vi "WriteXML.vi"(8 "error in (no error)":errorcluster, 10 "Path":path, 11 "PixelflySettings in":refnum<class "PixelflySettings.lvclass">) -> (0 "error out":errorcluster, 3 "PixelflySettings out":refnum<class "PixelflySettings.lvclass">)   [LabVIEW 2011, in "Tools.lvlib" / "Settings.lvlib" / "PixelflySettings.lvclass"]
uses:
  PixelflySettings.lvclass
  NativeXML/NativeXML.lvclass
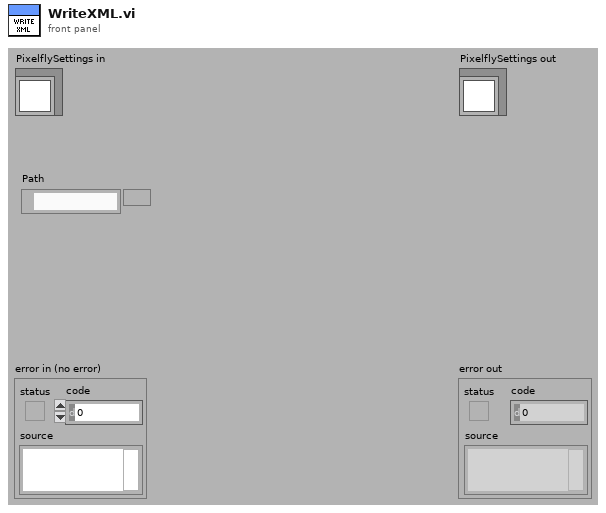
[diagram p1: front panel]
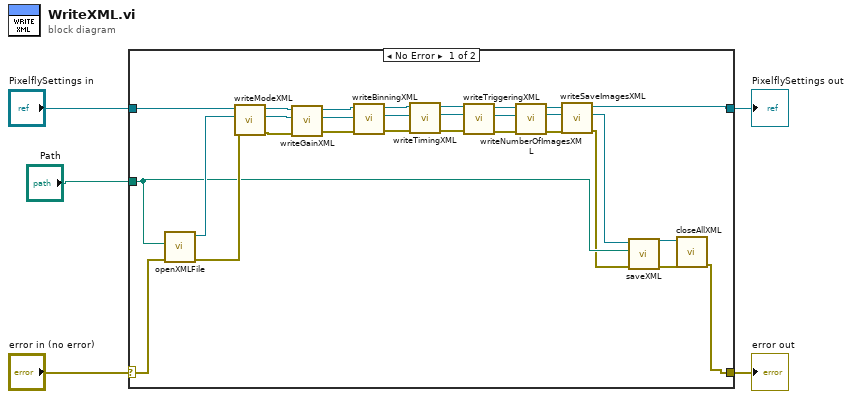
[diagram p0: block diagram]
diagram:
  n1 = case shown="No Error" "error in (no error)" {
    selector: "error in (no error)" -> [w19 w36]
    tunnel: [w15 w36] -> w4
    tunnel: [w8 w35] -> w2
    tunnel: "PixelflySettings in" -> [w34 w35]
    tunnel: "Path" -> [w18 _]
    frame No Error {
      n2 = call "openXMLFile.vi"("error in (no error)"=w19, "Path"=w18) -> ("error out"=w20:errorcluster, "NativeXML out"=w21:refnum<class "NativeXML.lvclass">)  [unwired: 8 in]
      n3 = call "writeModeXML.vi"("error in (no error)"=w20, "NativeXML in"=w21, "PixelflySettings in"=w34) -> ("error out"=w22:errorcluster, "NativeXML out"=w29:refnum<class "NativeXML.lvclass">, "PixelflySettings out"=w33:refnum<class "PixelflySettings.lvclass">)  [unwired: 6 in]
      n4 = call "writeGainXML.vi"("error in (no error)"=w22, "NativeXML in"=w29, "PixelflySettings in"=w33) -> ("error out"=w23:errorcluster, "NativeXML out"=w28:refnum<class "NativeXML.lvclass">, "PixelflySettings out"=w32:refnum<class "PixelflySettings.lvclass">)  [unwired: 6 in]
      n5 = call "writeBinningXML.vi"("error in (no error)"=w23, "NativeXML in"=w28, "PixelflySettings in"=w32) -> ("error out"=w24:errorcluster, "NativeXML out"=w27:refnum<class "NativeXML.lvclass">, "PixelflySettings out"=w31:refnum<class "PixelflySettings.lvclass">)  [unwired: 6 in]
      n6 = call "writeTimingXML.vi"("error in (no error)"=w24, "NativeXML in"=w27, "PixelflySettings in"=w31) -> ("error out"=w25:errorcluster, "NativeXML out"=w26:refnum<class "NativeXML.lvclass">, "PixelflySettings out"=w30:refnum<class "PixelflySettings.lvclass">)  [unwired: 6 in]
      n7 = call "writeTriggeringXML.vi"("error in (no error)"=w25, "NativeXML in"=w26, "PixelflySettings in"=w30) -> ("error out"=w14:errorcluster, "NativeXML out"=w13:refnum<class "NativeXML.lvclass">, "PixelflySettings out"=w12:refnum<class "PixelflySettings.lvclass">)  [unwired: 6 in]
      n8 = call "writeNumberOfImagesXML.vi"("error in (no error)"=w14, "NativeXML in"=w13, "PixelflySettings in"=w12) -> ("error out"=w9:errorcluster, "NativeXML out"=w10:refnum<class "NativeXML.lvclass">, "PixelflySettings out"=w11:refnum<class "PixelflySettings.lvclass">)  [unwired: 6 in]
      n9 = call "writeSaveImagesXML.vi"("error in (no error)"=w9, "NativeXML in"=w10, "PixelflySettings in"=w11) -> ("error out"=w6:errorcluster, "NativeXML out"=w7:refnum<class "NativeXML.lvclass">, "PixelflySettings out"=w8:refnum<class "PixelflySettings.lvclass">)  [unwired: 6 in]
      n10 = call "saveXML.vi"("error in (no error)"=w6, "Path"=w18, "NativeXML in"=w7) -> ("error out"=w17:errorcluster, "NativeXML out"=w16:refnum<class "NativeXML.lvclass">)  [unwired: 7 in]
      n11 = call "closeAllXML.vi"("error in (no error)"=w17, "NativeXML in"=w16) -> ("error out"=w15:errorcluster)  [unwired: 9 in]
    }
    frame Error {
    }
  }
  "error out" <- w4
  "PixelflySettings out" <- w2
